vi "Update Flags To Server.vi"(8 "error in":errorcluster, 10 "Selected Flag":i32, 11 "State Cluster":T1) -> (0 "error out":errorcluster)   [LabVIEW 2015]
uses:
  TypeDef/State Cluster.ctl
  LVClasses/Room/Room.lvclass
  LVClasses/Room/Room.lvclass/Room.ctl
  LVClasses/Flags/Flags.lvclass/Flags.ctl
  LVClasses/Room/Read Flags.lvclass.vi
  LVClasses/Room/Read Room Number.vi
  LVClasses/Flags/Read State.vi
  LVClasses/Flags/Flags.lvclass
  LVRestAPI/RoomRestApi.lvlib
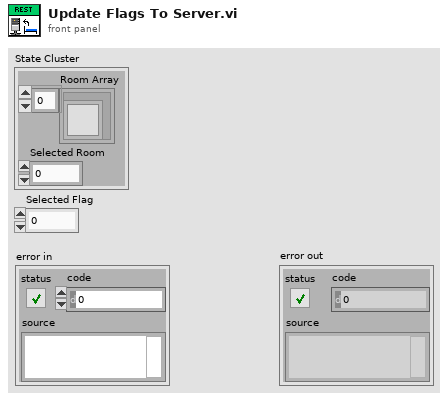
[diagram p1: front panel]
types:
  T1 = typedef "State Cluster.ctl" = cluster{"Room Array":refnum<class "Room.lvclass">[], "Selected Room":u32}
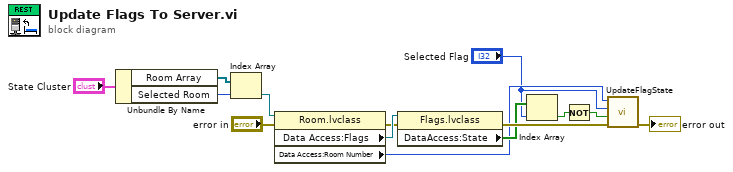
[diagram p0: block diagram]
diagram:
  n1 = Unbundle By Name("State Cluster") -> ("Room Array"=w12:refnum<class "Room.lvclass">[], "Selected Room"=w13:u32)
  n2 = Index Array(array=w12, index=w13) -> (element=w11:refnum<class "Room.lvclass">)
  n3 = property class="Room.lvclass"(reference=w11, error in="error in") -> (error out=w9:errorcluster, "Data Access:Flags"=w10:refnum<class "Flags.lvclass">, "Data Access:Room Number"=w5:i32)  [unwired: 1 out]
  n4 = property class="Flags.lvclass"(reference=w10, error in=w9) -> (error out=w7:errorcluster, "DataAccess:State"=w6:bool[])  [unwired: 1 out]
  n5 = Index Array(array=w6, index="Selected Flag") -> (element=w2:bool)
  n6 = Not(x=w2) -> (.not. x?=w1:bool)
  n7 = call "UpdateFlagState.vi"("error in (no error)"=w7, "State"=w1, "Index"="Selected Flag", "Room Number"=w5) -> ("error out"=→"error out":errorcluster)  [unwired: 6 in, 1 out]
